vi "SimpleLiveAppWithROI.vi"() -> ()   [LabVIEW 2020]
uses:
  C:/Users/Public/Documents/Photometrics/PMQI-LabViewSamples/Examples/2018/Dependencies/PVCamNET.dll
  Dependencies/PVCamNET.dll
panel:
  in  "Full CCD":bool
  in  "Full CCD Height":u16
  in  "Full CCD Width":u16
  in  "Get ROI":bool
  in  "Height":u16
  in  "Y":u16
  in  "Width":u16
  in  "X":u16
  in  "Exposure Time [ms]":dbl
  in  "Live":bool
  in  "Camera Status":bool
  in  "Uninit":bool
  in  "Live stop":bool
  in  "Live start":bool
  in  "Init":bool
  # "SimpleLiveAppWithROI.vi\n\nDescription:\nThis sample code lets the user use live mode in an event driven structure.\nThe user can create a ROI from CamWindow and find out the coordinate.\n\nSteps to run:\n1. Click \"Run\"\n2. Click \"Open\"\n3. Enter Exposure Time\n4. Click \"Live start\"\n5. Click \"Live stop\"\n6. Right click on CamWindow and add a ROI.\n7. Click \"Get ROI\"\n8. Click \"Live start\"\n9. Click \"Live stop\"\n10. Right click on CamWindow and delete a ROI.\n11. Click \"Close\""
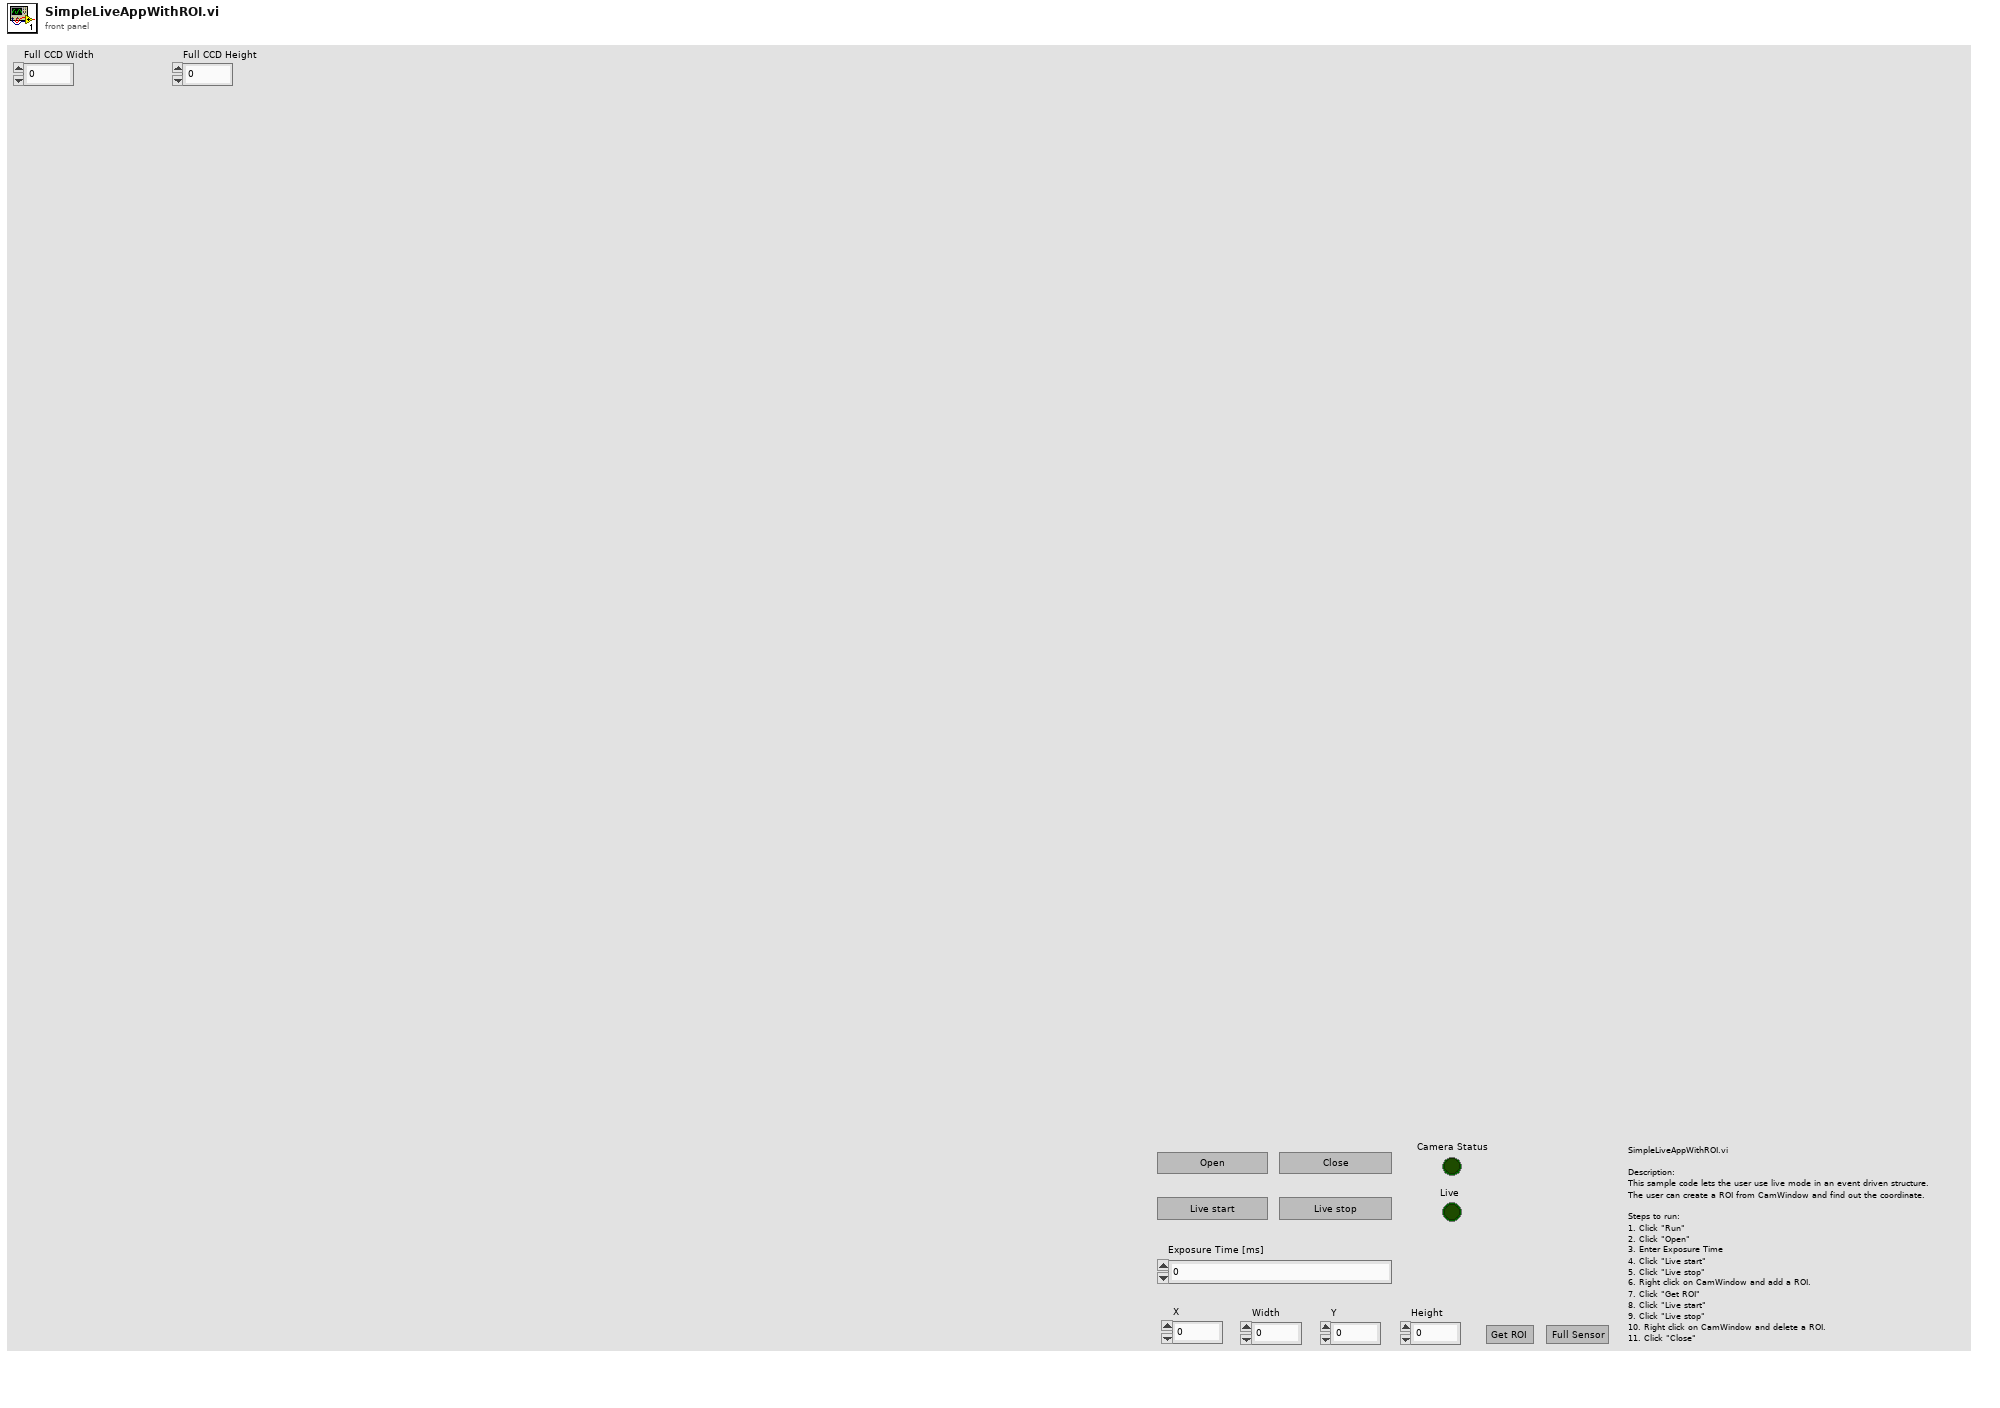
[diagram p1: front panel]
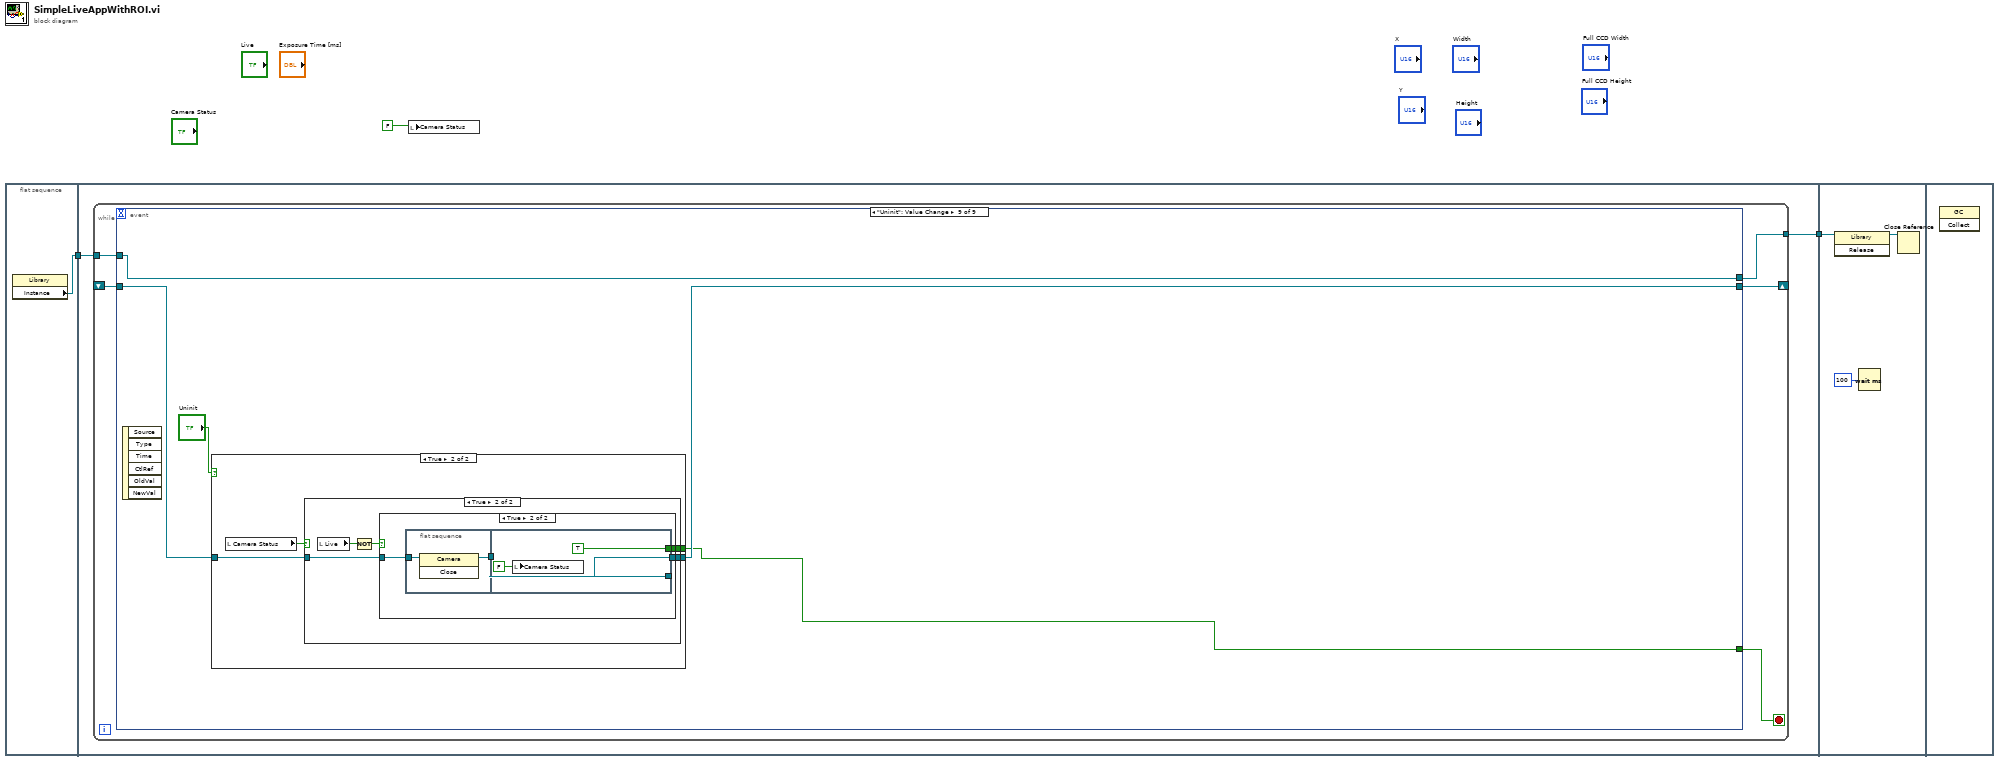
[diagram p0: block diagram]
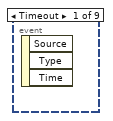
[diagram p2: hidden frame]
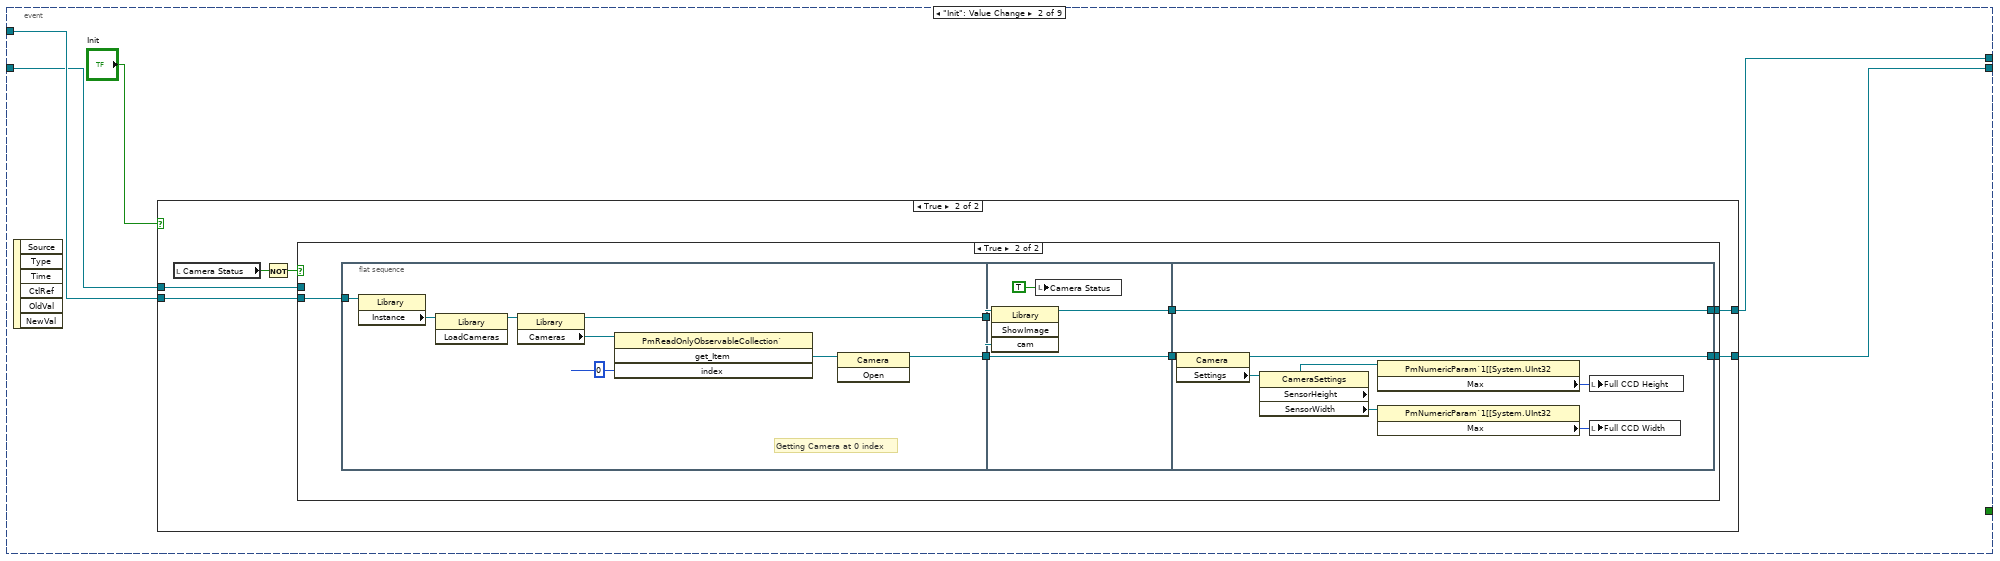
[diagram p3: hidden frame]
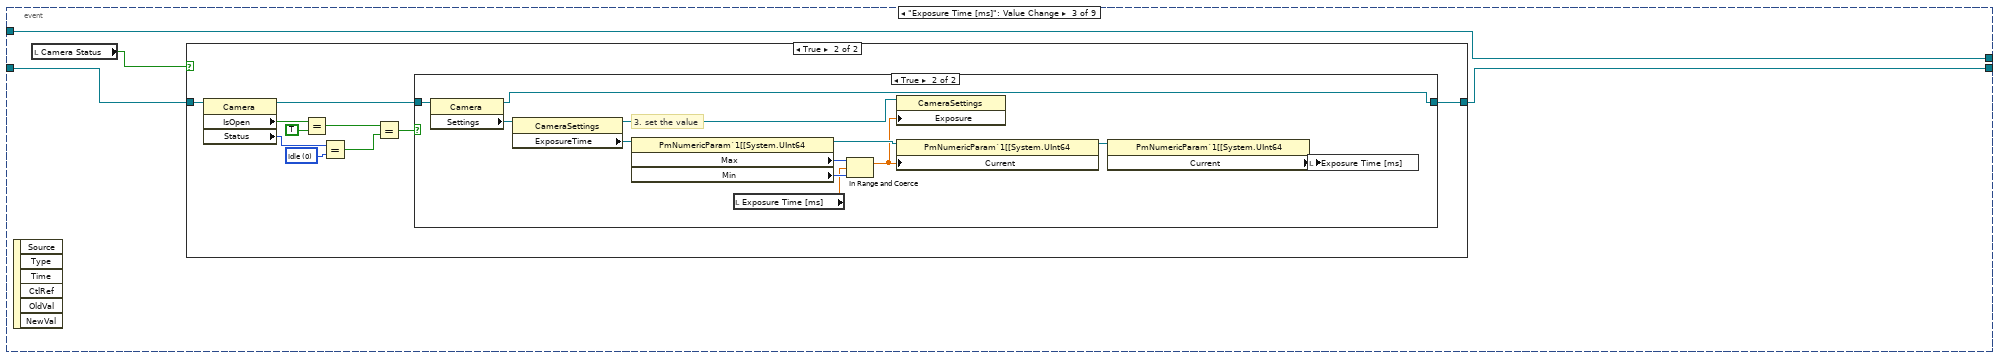
[diagram p6: hidden frame]
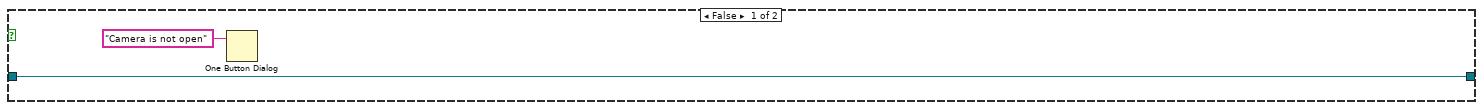
[diagram p7: hidden frame]
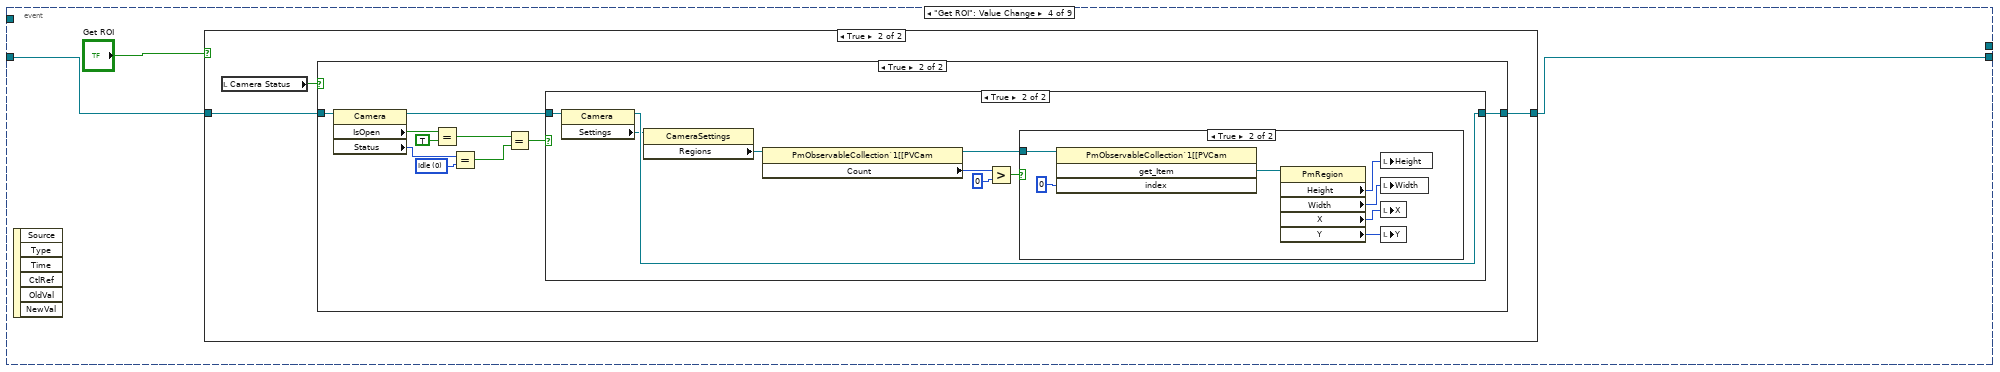
[diagram p9: hidden frame]
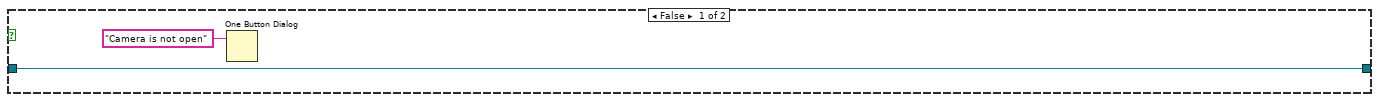
[diagram p11: hidden frame]
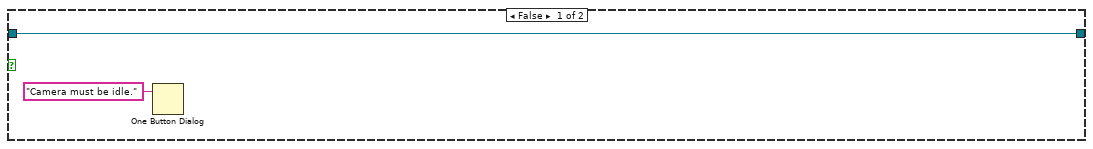
[diagram p12: hidden frame]
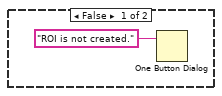
[diagram p13: hidden frame]
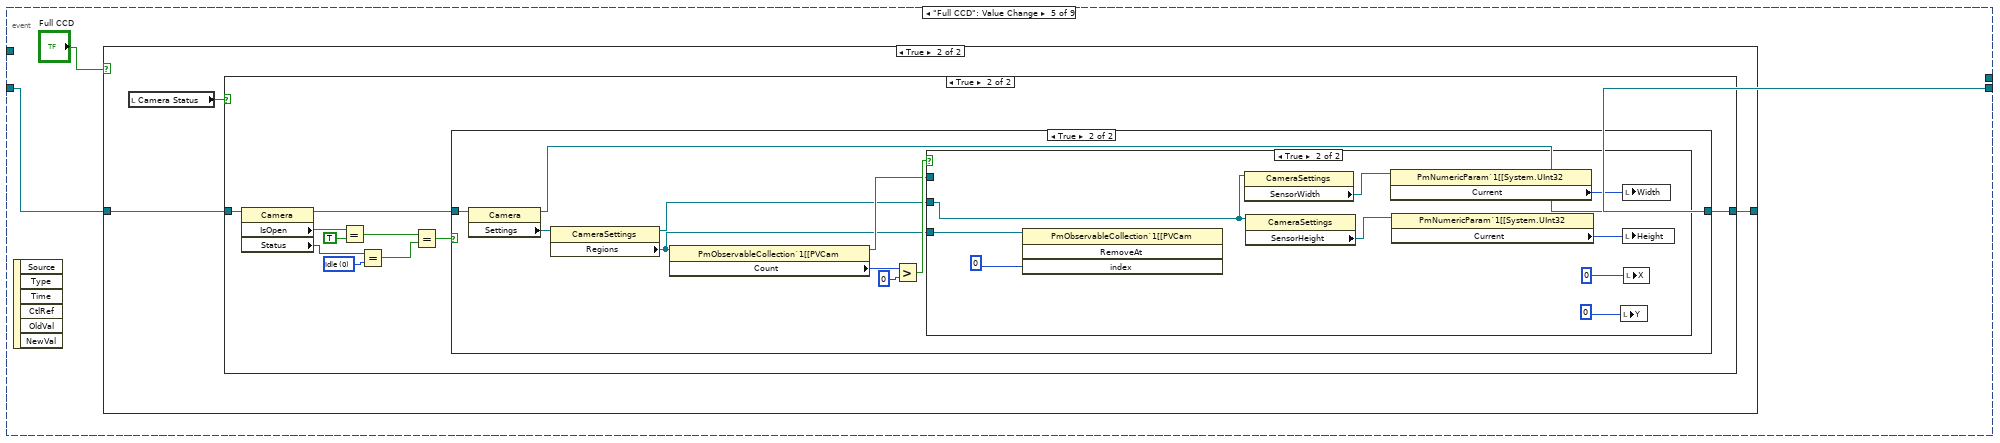
[diagram p14: hidden frame]
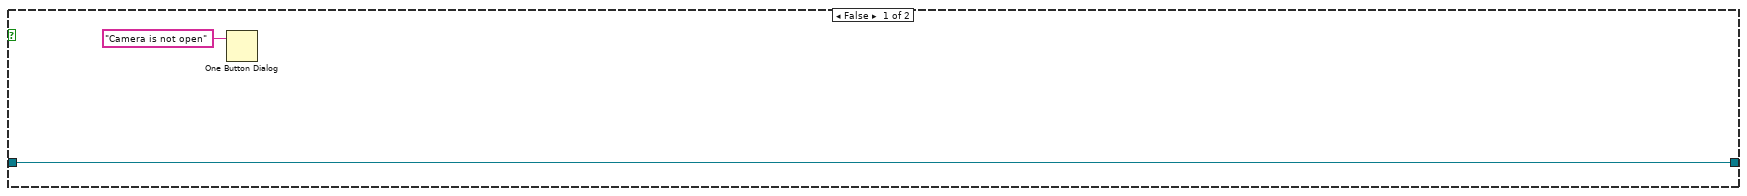
[diagram p16: hidden frame]
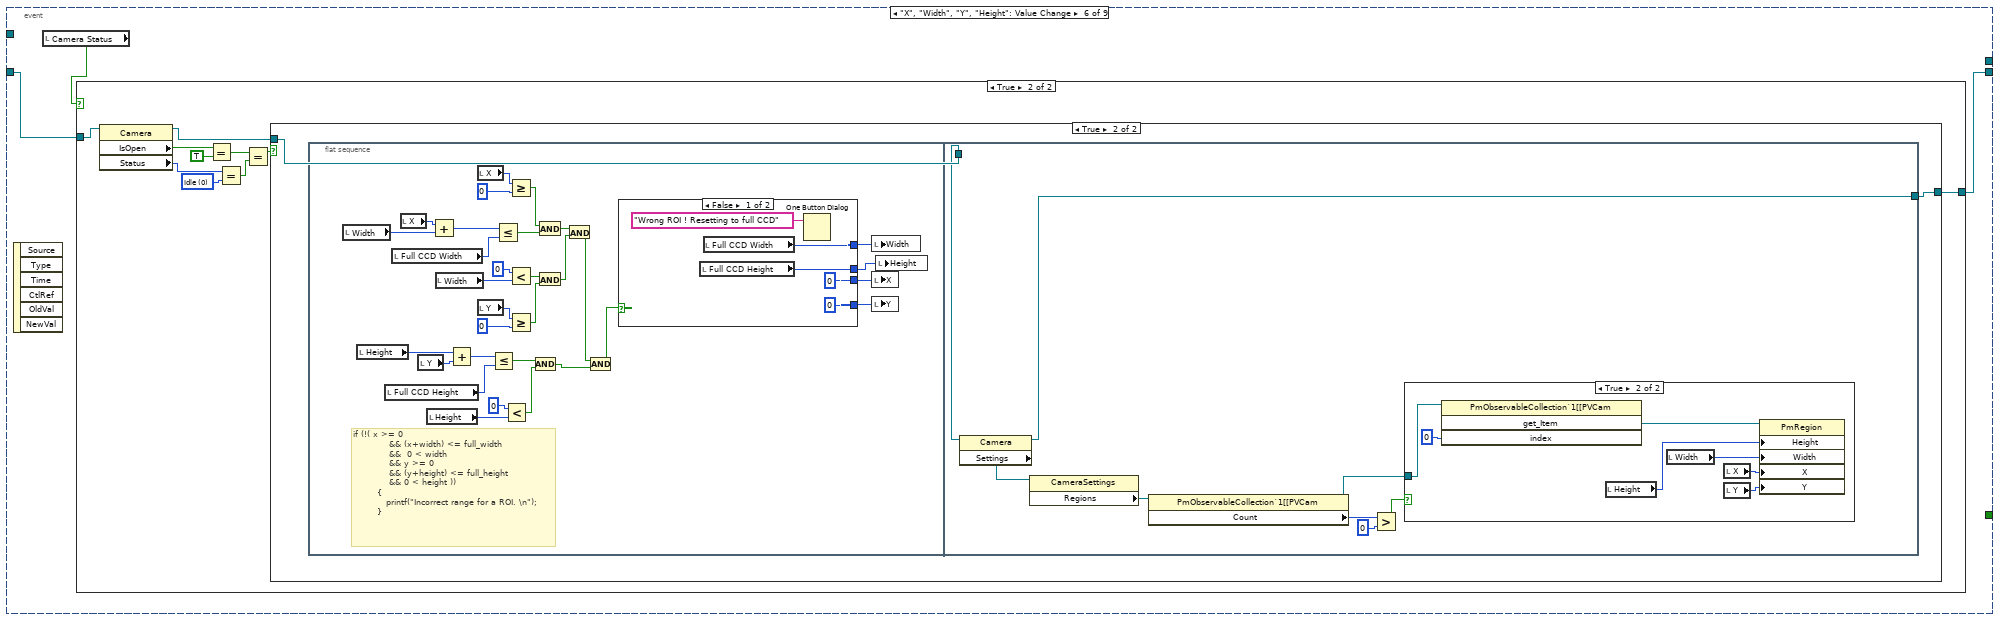
[diagram p19: hidden frame]
diagram:
  n1 = flat-sequence {
    tunnel: [w4] -> w3
    tunnel: w3 -> [w6]
    tunnel: [w5] -> w2
    tunnel: w2 -> [w314]
    frame #0 {
      n2 = property class="Library"() -> ("Instance"=w4:refnum<k24>)  [unwired: 2 in, 2 out]
    }
    frame #1 {
      n3 = while {
        tunnel: w6 -> [w11]
        shift-right: [w7] -> _
        shift-left: _ -> [w9]
        tunnel: [w10] -> w5
        stop <- w8 stop-if-true
        n4 = event shown="[8] \"Uninit\": Value Change" {
          selector: _ -> [_ _ _ _ _ _ _ _ _]
          dyn-events: _ -> [_ _ _ _ _ _ _ _ _]
          timeout: _ -> [_ _ _ _ _ _ _ _ _]
          tunnel: w11 -> [_ w16 w54 _ _ _ w231 _ w286]
          tunnel: [_ w15 w56 w83 w121 w159 w232 w261 w287] -> w7
          tunnel: [_ w14 w54 _ _ _ w231 _ w286] -> w10
          tunnel: w9 -> [_ w13 w57 w85 w122 w158 w233 w262 w288]
          tunnel: [_ _ _ _ _ _ _ _ w285] -> w8
          event Timeout {
            n5 = event-data() -> ()  [unwired: 1 in, 3 out]
          }
          event "Init": Value Change {
            n6 = event-data() -> ()  [unwired: 1 in, 6 out]
            n7 = case shown="True" "Init" {
              tunnel: w16 -> [w18 w24]
              tunnel: [w17 w23] -> w15
              tunnel: [w18 w22] -> w14
              tunnel: w13 -> [w17 w19]
              frame False {
              }
              frame True {
                n8 = local read "Camera Status"() -> (w21:bool)
                n9 = Not(x=w21) -> (.not. x?=w20:bool)
                n10 = case shown="True" w20 {
                  tunnel: w24 -> [w25 w31]
                  tunnel: [w26 w30] -> w23
                  tunnel: [w25 w29] -> w22
                  tunnel: w19 -> [w26 _]
                  frame False {
                  }
                  frame True {
                    n11 = flat-sequence {
                      tunnel: w31 -> [w36]
                      tunnel: [w38] -> w33
                      tunnel: [w37] -> w32
                      tunnel: w33 -> [w44]
                      tunnel: w32 -> [w45]
                      tunnel: [w45] -> w28
                      tunnel: [w43] -> w27
                      tunnel: [w53] -> w29
                      tunnel: [w48] -> w30
                      tunnel: w28 -> [w52]
                      tunnel: w27 -> [w53]
                      frame #0 {
                        # "Getting Camera at 0 index"
                        n12 = property class="Library"(reference=w36) -> ("Instance"=w35:refnum<k24>)  [unwired: 1 in, 2 out]
                        n13 = invoke class="Library" method="LoadCameras"(reference=w35) -> (reference out=w34:refnum<k24>)  [unwired: 2 in, 2 out]
                        n14 = property class="Library"(reference=w34) -> (reference out=w38:refnum<k24>, "Cameras"=w41:refnum<k24>)  [unwired: 1 in, 1 out]
                        n15 = invoke class="PmReadOnlyObservableCollection`" method="get_Item"(reference=w41, "index"=0) -> ("get_Item"=w39:refnum<k24>)  [unwired: 2 in, 3 out]
                        n16 = invoke class="Camera" method="Open"(reference=w39) -> (reference out=w37:refnum<k24>)  [unwired: 2 in, 2 out]
                      }
                      frame #1 {
                        n17 = invoke class="Library" method="ShowImage"(reference=w44, "cam"=w45) -> (reference out=w43:refnum<k24>)  [unwired: 2 in, 3 out]
                        n18 = local write "Camera Status"(TRUE ("Camera Status")) -> ()
                      }
                      frame #2 {
                        n19 = property class="Camera"(reference=w52) -> (reference out=w48:refnum<k24>, "Settings"=w51:refnum<k24>)  [unwired: 1 in, 1 out]
                        n20 = property class="CameraSettings"(reference=w51) -> ("SensorHeight"=w50:refnum<k24>, "SensorWidth"=w49:refnum<k24>)  [unwired: 1 in, 2 out]
                        n21 = property class="PmNumericParam`1[[System.UInt32"(reference=w50) -> ("Max"=w47:u32)  [unwired: 1 in, 2 out]
                        n22 = property class="PmNumericParam`1[[System.UInt32"(reference=w49) -> ("Max"=w46:u32)  [unwired: 1 in, 2 out]
                        n23 = local write "Full CCD Height"(w47) -> ()
                        n24 = local write "Full CCD Width"(w46) -> ()
                      }
                    }
                  }
                }
              }
            }
          }
          event "Exposure Time [ms]": Value Change {
            n25 = event-data() -> ()  [unwired: 1 in, 6 out]
            n26 = local read "Camera Status"() -> (w55:bool)
            n27 = case shown="True" w55 {
              tunnel: w57 -> [w59 w63]
              tunnel: [w59 w60] -> w56
              frame False {
                n28 = One Button Dialog(message="Camera is not open") -> ()  [unwired: 1 in, 1 out]
              }
              frame True {
                w68 = 0 items=["Idle", "Capturing"] ("Status")
                n29 = property class="Camera"(reference=w63) -> (reference out=w61:refnum<k24>, "IsOpen"=w67:bool, "Status"=w69:i32)  [unwired: 1 in, 1 out]
                n30 = Equal?(x=w67, y=TRUE) -> (x = y?=w65:bool)
                n31 = Equal?(x=w69, y=w68) -> (x = y?=w64:bool)
                n32 = Equal?(x=w65, y=w64) -> (x = y?=w62:bool)
                n33 = case shown="True" w62 {
                  tunnel: w61 -> [w70 w82]
                  tunnel: [w70 w71] -> w60
                  frame False {
                  }
                  frame True {
                    # "3. set the value"
                    n34 = property class="Camera"(reference=w82) -> (reference out=w71:refnum<k24>, "Settings"=w81:refnum<k24>)  [unwired: 1 in, 1 out]
                    n35 = property class="CameraSettings"(reference=w81) -> (reference out=w74:refnum<k24>, "ExposureTime"=w75:refnum<k24>)  [unwired: 1 in, 1 out]
                    n36 = property class="PmNumericParam`1[[System.UInt64"(reference=w75) -> (reference out=w78:refnum<k24>, "Max"=w80:u64, "Min"=w79:u64)  [unwired: 1 in, 1 out]
                    n37 = local read "Exposure Time [ms]"() -> (w73:dbl)
                    n38 = In Range and Coerce(upper limit=w80, x=w73, lower limit=w79) -> (coerced(x)=w76:dbl)  [unwired: 1 out]
                    n39 = property class="CameraSettings"(reference=w74, "Exposure"=w76) -> ()  [unwired: 1 in, 2 out]
                    n40 = property class="PmNumericParam`1[[System.UInt64"(reference=w78, "Current"=w76) -> (reference out=w77:refnum<k24>)  [unwired: 1 in, 1 out]
                    n41 = property class="PmNumericParam`1[[System.UInt64"(reference=w77) -> ("Current"=w72:u64)  [unwired: 1 in, 2 out]
                    n42 = local write "Exposure Time [ms]"(w72) -> ()
                  }
                }
              }
            }
          }
          event "Get ROI": Value Change {
            n43 = event-data() -> ()  [unwired: 1 in, 6 out]
            n44 = case shown="True" "Get ROI" {
              tunnel: w85 -> [w86 w89]
              tunnel: [w86 w88] -> w83
              frame False {
              }
              frame True {
                n45 = local read "Camera Status"() -> (w87:bool)
                n46 = case shown="True" w87 {
                  tunnel: w89 -> [w91 w95]
                  tunnel: [w91 w92] -> w88
                  frame False {
                    n47 = One Button Dialog(message="Camera is not open") -> ()  [unwired: 1 in, 1 out]
                  }
                  frame True {
                    w100 = 0 items=["Idle", "Capturing"] ("Status")
                    n48 = property class="Camera"(reference=w95) -> (reference out=w94:refnum<k24>, "IsOpen"=w99:bool, "Status"=w101:i32)  [unwired: 1 in, 1 out]
                    n49 = Equal?(x=w99, y=TRUE) -> (x = y?=w97:bool)
                    n50 = Equal?(x=w101, y=w100) -> (x = y?=w96:bool)
                    n51 = Equal?(x=w97, y=w96) -> (x = y?=w93:bool)
                    n52 = case shown="True" w93 {
                      tunnel: w94 -> [w103 w111]
                      tunnel: [w103 w110] -> w92
                      frame False {
                        n53 = One Button Dialog(message="Camera must be idle.") -> ()  [unwired: 1 in, 1 out]
                      }
                      frame True {
                        n54 = property class="Camera"(reference=w111) -> (reference out=w110:refnum<k24>, "Settings"=w109:refnum<k24>)  [unwired: 1 in, 1 out]
                        n55 = property class="CameraSettings"(reference=w109) -> ("Regions"=w108:refnum<k24>)  [unwired: 1 in, 2 out]
                        n56 = property class="PmObservableCollection`1[[PVCam"(reference=w108) -> (reference out=w104:refnum<k24>, "Count"=w107:i32)  [unwired: 1 in, 1 out]
                        n57 = Greater?(x=w107, y=0) -> (0:w105:bool)
                        n58 = case shown="True" w105 {
                          tunnel: w104 -> [_ w113]
                          frame False {
                            n59 = One Button Dialog(message="ROI is not created.") -> ()  [unwired: 1 in, 1 out]
                          }
                          frame True {
                            n60 = invoke class="PmObservableCollection`1[[PVCam" method="get_Item"(reference=w113, "index"=0) -> ("get_Item"=w119:refnum<k24>)  [unwired: 2 in, 3 out]
                            n61 = property class="PmRegion"(reference=w119) -> ("Height"=w117:u16, "Width"=w116:u16, "X"=w115:u16, "Y"=w114:u16)  [unwired: 1 in, 2 out]
                            n62 = local write "Height"(w117) -> ()
                            n63 = local write "Width"(w116) -> ()
                            n64 = local write "X"(w115) -> ()
                            n65 = local write "Y"(w114) -> ()
                          }
                        }
                      }
                    }
                  }
                }
              }
            }
          }
          event "Full CCD": Value Change {
            n66 = event-data() -> ()  [unwired: 1 in, 6 out]
            n67 = case shown="True" "Full CCD" {
              tunnel: w122 -> [w123 w126]
              tunnel: [w123 w125] -> w121
              frame False {
              }
              frame True {
                n68 = local read "Camera Status"() -> (w124:bool)
                n69 = case shown="True" w124 {
                  tunnel: w126 -> [w128 w132]
                  tunnel: [w128 w129] -> w125
                  frame False {
                    n70 = One Button Dialog(message="Camera is not open") -> ()  [unwired: 1 in, 1 out]
                  }
                  frame True {
                    w137 = 0 items=["Idle", "Capturing"] ("Status")
                    n71 = property class="Camera"(reference=w132) -> (reference out=w131:refnum<k24>, "IsOpen"=w136:bool, "Status"=w138:i32)  [unwired: 1 in, 1 out]
                    n72 = Equal?(x=w136, y=TRUE) -> (x = y?=w134:bool)
                    n73 = Equal?(x=w138, y=w137) -> (x = y?=w133:bool)
                    n74 = Equal?(x=w134, y=w133) -> (x = y?=w130:bool)
                    n75 = case shown="True" w130 {
                      tunnel: w131 -> [w139 w148]
                      tunnel: [w139 w147] -> w129
                      frame False {
                      }
                      frame True {
                        n76 = property class="Camera"(reference=w148) -> (reference out=w147:refnum<k24>, "Settings"=w146:refnum<k24>)  [unwired: 1 in, 1 out]
                        n77 = property class="CameraSettings"(reference=w146) -> (reference out=w140:refnum<k24>, "Regions"=w141:refnum<k24>)  [unwired: 1 in, 1 out]
                        n78 = property class="PmObservableCollection`1[[PVCam"(reference=w141) -> (reference out=w142:refnum<k24>, "Count"=w145:i32)  [unwired: 1 in, 1 out]
                        n79 = Greater?(x=w145, y=0) -> (0:w143:bool)
                        n80 = case shown="True" w143 {
                          tunnel: w142 -> [_ _]
                          tunnel: w141 -> [_ w157]
                          tunnel: w140 -> [_ w151]
                          frame False {
                          }
                          frame True {
                            n81 = invoke class="PmObservableCollection`1[[PVCam" method="RemoveAt"(reference=w157, "index"=0) -> ()  [unwired: 2 in, 4 out]
                            n82 = property class="CameraSettings"(reference=w151) -> ("SensorWidth"=w153:refnum<k24>)  [unwired: 1 in, 2 out]
                            n83 = property class="CameraSettings"(reference=w151) -> ("SensorHeight"=w154:refnum<k24>)  [unwired: 1 in, 2 out]
                            n84 = property class="PmNumericParam`1[[System.UInt32"(reference=w153) -> ("Current"=w152:u32)  [unwired: 1 in, 2 out]
                            n85 = property class="PmNumericParam`1[[System.UInt32"(reference=w154) -> ("Current"=w155:u32)  [unwired: 1 in, 2 out]
                            n86 = local write "Y"(0 ("index")) -> ()
                            n87 = local write "Width"(w152) -> ()
                            n88 = local write "Height"(w155) -> ()
                            n89 = local write "X"(0 ("index")) -> ()
                          }
                        }
                      }
                    }
                  }
                }
              }
            }
          }
          event "X", "Width", "Y", "Height": Value Change {
            n90 = event-data() -> ()  [unwired: 1 in, 6 out]
            n91 = local read "Camera Status"() -> (w160:bool)
            n92 = case shown="True" w160 {
              tunnel: w158 -> [w161 w164]
              tunnel: [w161 w162] -> w159
              frame False {
              }
              frame True {
                w170 = 0 items=["Idle", "Capturing"] ("Status")
                n93 = property class="Camera"(reference=w164) -> (reference out=w163:refnum<k24>, "IsOpen"=w169:bool, "Status"=w171:i32)  [unwired: 1 in, 1 out]
                n94 = Equal?(x=w169, y=TRUE) -> (x = y?=w167:bool)
                n95 = Equal?(x=w171, y=w170) -> (x = y?=w166:bool)
                n96 = Equal?(x=w167, y=w166) -> (x = y?=w165:bool)
                n97 = case shown="True" w165 {
                  tunnel: w163 -> [w172 w174]
                  tunnel: [w172 w173] -> w162
                  frame False {
                  }
                  frame True {
                    n98 = flat-sequence {
                      tunnel: w174 -> [w222]
                      tunnel: [w221] -> w173
                      frame #0 {
                        # "if (!( x >= 0\n            && (x+width) <= full_width\n            &&  0 < width \n            && y >= 0\n            && (y+height) <= full_height\n            && 0 < height ))\n        {\n           printf(\"Incorrect range for a ROI. \\n\");\n        }"
                        n99 = local read "Width"() -> (w190:u16)
                        n100 = local read "Height"() -> (w188:u16)
                        n101 = local read "Full CCD Height"() -> (w184:u16)
                        n102 = local read "Full CCD Width"() -> (w186:u16)
                        n103 = local read "X"() -> (w191:u16)
                        n104 = local read "Y"() -> (w187:u16)
                        n105 = local read "Height"() -> (w179:u16)
                        n106 = Add(x=w191, y=w190) -> (x+y=w185:u16)
                        n107 = local read "Width"() -> (w182:u16)
                        n108 = Add(x=w188, y=w187) -> (x+y=w183:u16)
                        n109 = local read "X"() -> (w192:u16)
                        n110 = local read "Y"() -> (w189:u16)
                        n111 = Less Or Equal?(x=w183, y=w184) -> (x <= y?=w199:bool)
                        n112 = Less Or Equal?(x=w185, y=w186) -> (x <= y?=w202:bool)
                        n113 = Less?(x=u16 0 ("y"), y=w179) -> (x < y?=w198:bool)
                        n114 = Greater Or Equal?(x=w192, y=u16 0) -> (x >= y?=w203:bool)
                        n115 = Less?(x=u16 0 ("y"), y=w182) -> (x < y?=w201:bool)
                        n116 = Greater Or Equal?(x=w189, y=u16 0) -> (x >= y?=w200:bool)
                        n117 = And(x=w199, y=w198) -> (x .and. y?=w194:bool)
                        n118 = And(x=w203, y=w202) -> (x .and. y?=w197:bool)
                        n119 = And(x=w201, y=w200) -> (x .and. y?=w196:bool)
                        n120 = And(x=w197, y=w196) -> (x .and. y?=w195:bool)
                        n121 = And(x=w195, y=w194) -> (x .and. y?=w193:bool)
                        n122 = case shown="False" w193 {
                          tunnel: [w207 w214] -> w178
                          tunnel: [u16 0 ("X") w213] -> w175
                          tunnel: [u16 0 ("Y") w212] -> w176
                          tunnel: [w208 w211] -> w177
                          frame False {
                            n123 = local read "Full CCD Height"() -> (w208:u16)
                            n124 = local read "Full CCD Width"() -> (w207:u16)
                            n125 = One Button Dialog(message="Wrong ROI ! Resetting to full CCD") -> ()  [unwired: 1 in, 1 out]
                          }
                          frame True {
                            n126 = local read "Height"() -> (w211:u16)
                            n127 = local read "Width"() -> (w214:u16)
                            n128 = local read "X"() -> (w213:u16)
                            n129 = local read "Y"() -> (w212:u16)
                          }
                        }
                        n130 = local write "Width"(w178) -> ()
                        n131 = local write "X"(w175) -> ()
                        n132 = local write "Y"(w176) -> ()
                        n133 = local write "Height"(w177) -> ()
                      }
                      frame #1 {
                        n134 = property class="Camera"(reference=w222) -> (reference out=w221:refnum<k24>, "Settings"=w220:refnum<k24>)  [unwired: 1 in, 1 out]
                        n135 = property class="CameraSettings"(reference=w220) -> ("Regions"=w219:refnum<k24>)  [unwired: 1 in, 2 out]
                        n136 = property class="PmObservableCollection`1[[PVCam"(reference=w219) -> (reference out=w215:refnum<k24>, "Count"=w218:i32)  [unwired: 1 in, 1 out]
                        n137 = Greater?(x=w218, y=0) -> (0:w216:bool)
                        n138 = case shown="True" w216 {
                          tunnel: w215 -> [_ w228]
                          frame False {
                            n139 = One Button Dialog(message="ROI is not created.") -> ()  [unwired: 1 in, 1 out]
                          }
                          frame True {
                            n140 = invoke class="PmObservableCollection`1[[PVCam" method="get_Item"(reference=w228, "index"=0) -> ("get_Item"=w230:refnum<k24>)  [unwired: 2 in, 3 out]
                            n141 = local read "Height"() -> (w227:u16)
                            n142 = local read "Width"() -> (w226:u16)
                            n143 = local read "X"() -> (w225:u16)
                            n144 = local read "Y"() -> (w224:u16)
                            n145 = property class="PmRegion"(reference=w230, "Height"=w227, "Width"=w226, "X"=w225, "Y"=w224) -> ()  [unwired: 1 in, 2 out]
                          }
                        }
                      }
                    }
                  }
                }
              }
            }
          }
          event "Live start": Value Change {
            n146 = event-data() -> ()  [unwired: 1 in, 6 out]
            n147 = case shown="True" "Live start" {
              tunnel: w233 -> [w235 w238]
              tunnel: [w235 w237] -> w232
              frame False {
              }
              frame True {
                n148 = local read "Camera Status"() -> (w236:bool)
                n149 = case shown="True" w236 {
                  tunnel: w238 -> [w239 w244]
                  tunnel: [w239 w242] -> w237
                  frame False {
                    n150 = One Button Dialog(message="Camera is not open") -> ()  [unwired: 1 in, 1 out]
                  }
                  frame True {
                    w249 = 0 items=["Idle", "Capturing"] ("Status")
                    n151 = property class="Camera"(reference=w244) -> (reference out=w243:refnum<k24>, "IsOpen"=w248:bool, "Status"=w250:i32)  [unwired: 1 in, 1 out]
                    n152 = Equal?(x=w248, y=TRUE) -> (x = y?=w246:bool)
                    n153 = Equal?(x=w250, y=w249) -> (x = y?=w245:bool)
                    n154 = Equal?(x=w246, y=w245) -> (x = y?=w241:bool)
                    n155 = case shown="True" w241 {
                      tunnel: w243 -> [w252 w254]
                      tunnel: [w252 w255] -> w242
                      frame False {
                        n156 = local write "Live"(FALSE ("Live 2")) -> ()
                      }
                      frame True {
                        n157 = flat-sequence {
                          tunnel: w254 -> [w260]
                          tunnel: [w257] -> w253
                          frame #0 {
                            n158 = property class="Camera"(reference=w260) -> (reference out=w257:refnum<k24>, "AcquisitionBuffer"=w259:refnum<k24>)  [unwired: 1 in, 1 out]
                            n159 = property class="AcqBuffer"(reference=w259, "BufferSize"=100) -> ()  [unwired: 1 in, 2 out]
                          }
                        }
                        n160 = local write "Live"(TRUE ("Live")) -> ()
                        n161 = invoke class="Camera" method="StartLive"(reference=w253) -> (reference out=w255:refnum<k24>)  [unwired: 2 in, 2 out]
                      }
                    }
                  }
                }
              }
            }
          }
          event "Live stop": Value Change {
            n162 = event-data() -> ()  [unwired: 1 in, 6 out]
            n163 = case shown="True" "Live stop" {
              tunnel: w262 -> [w264 w267]
              tunnel: [w264 w266] -> w261
              frame False {
              }
              frame True {
                n164 = local read "Camera Status"() -> (w265:bool)
                n165 = case shown="False" w265 {
                  tunnel: w267 -> [w269 w279]
                  tunnel: [w269 w276] -> w266
                  frame False {
                    n166 = One Button Dialog(message="Camera is not open") -> ()  [unwired: 1 in, 1 out]
                  }
                  frame True {
                    w274 = 1 items=["Idle", "Capturing"] ("Status")
                    n167 = property class="Camera"(reference=w279) -> (reference out=w277:refnum<k24>, "IsOpen"=w273:bool, "Status"=w275:i32)  [unwired: 1 in, 1 out]
                    n168 = Equal?(x=w275, y=w274) -> (x = y?=w270:bool)
                    n169 = Equal?(x=w273, y=TRUE) -> (x = y?=w271:bool)
                    n170 = Equal?(x=w271, y=w270) -> (x = y?=w278:bool)
                    n171 = case shown="True" w278 {
                      tunnel: w277 -> [w280 w283]
                      tunnel: [w280 w282] -> w276
                      frame False {
                      }
                      frame True {
                        n172 = invoke class="Camera" method="Stop"(reference=w283) -> (reference out=w282:refnum<k24>)  [unwired: 2 in, 2 out]
                        n173 = local write "Live"(FALSE ("Live 2")) -> ()
                      }
                    }
                  }
                }
              }
            }
          }
          event "Uninit": Value Change {
            n174 = event-data() -> ()  [unwired: 1 in, 6 out]
            n175 = case shown="True" "Uninit" {
              tunnel: w288 -> [w290 w294]
              tunnel: [w290 w293] -> w287
              tunnel: [FALSE ("Camera Status") w291] -> w285
              frame False {
              }
              frame True {
                n176 = local read "Camera Status"() -> (w292:bool)
                n177 = case shown="True" w292 {
                  tunnel: w294 -> [w296 w301]
                  tunnel: [w296 w300] -> w293
                  tunnel: [FALSE ("Camera Status") w299] -> w291
                  frame False {
                  }
                  frame True {
                    n178 = local read "Live"() -> (w297:bool)
                    n179 = Not(x=w297) -> (.not. x?=w298:bool)
                    n180 = case shown="True" w298 {
                      tunnel: w301 -> [w303 w306]
                      tunnel: [w303 w305] -> w300
                      tunnel: [FALSE ("Camera Status") w304] -> w299
                      frame False {
                      }
                      frame True {
                        n181 = flat-sequence {
                          tunnel: w306 -> [w309]
                          tunnel: [w308] -> w307
                          tunnel: [w312] -> w305
                          tunnel: w307 -> [w312]
                          tunnel: [TRUE ("Camera Status")] -> w304
                          frame #0 {
                            n182 = invoke class="Camera" method="Close"(reference=w309) -> (reference out=w308:refnum<k24>)  [unwired: 2 in, 2 out]
                          }
                          frame #1 {
                            n183 = local write "Camera Status"(FALSE ("Camera Status")) -> ()
                          }
                        }
                      }
                    }
                  }
                }
              }
            }
          }
        }
      }
    }
    frame #2 {
      n184 = invoke class="Library" method="Release"(reference=w314) -> (reference out=w315:refnum<k24>)  [unwired: 2 in, 2 out]
      n185 = Wait (ms)(milliseconds to wait=u32 100) -> ()  [unwired: 1 out]
      n186 = Close Reference(reference=w315) -> ()  [unwired: 1 in, 1 out]
    }
    frame #3 {
      n187 = invoke class="GC" method="Collect"() -> ()  [unwired: 3 in, 3 out]
    }
  }
  n188 = local write "Camera Status"(FALSE ("Camera Status")) -> ()
